vi "DHE_ParseAutoshutterCmd.vi"(8 "error in (no error)":errorcluster, 10 "argument":string, 11 "fd":i32) -> (0 "error out":errorcluster, 1 "ON?":bool, 2 "return value":i32, 3 "fd out":i32)   [LabVIEW 2016]
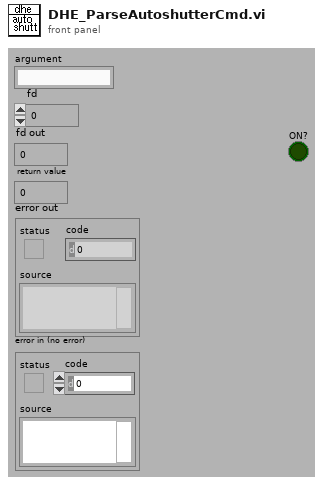
[diagram p1: front panel]
types:
  T1 = typedef "CMN_ContStatus.ctl" = cluster{"Response":string, "power":bool, "shutter":bool, "artifdata":bool, "idlemode":bool, "reset":bool, "gain":u8, "speed":u8, "resetPCI":bool, "autoshutter":bool, "TempSetPoint":i32, "multipleextensions":bool, "displayImage":bool, "coadding":bool, "images being coadded":i32, "Operation Mode":enum16{"normal", "coadd", "fawler"}, "frames to write":cluster{"subs":bool, "reset":bool, "exposed":bool}, "fawler samples":i32, "write auto":bool, "datatype":string, "frames to display":cluster{"subs":bool, "reset":bool, "exposed":bool}, "sur":i32, "autoclear":bool}
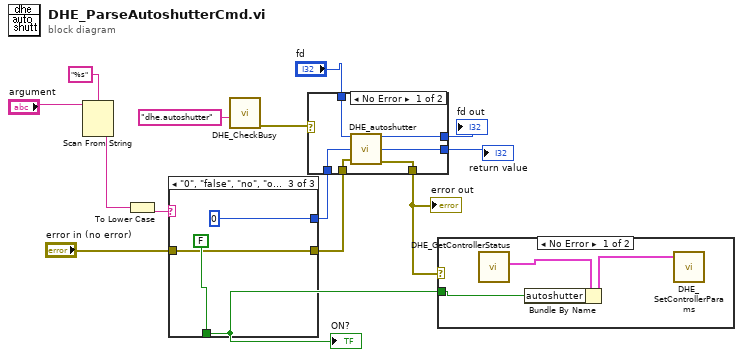
[diagram p0: block diagram]
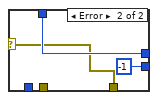
[diagram p2: hidden frame]
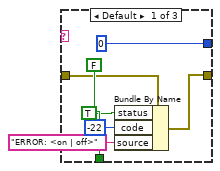
[diagram p4: hidden frame]
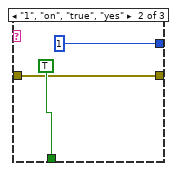
[diagram p5: hidden frame]
diagram:
  n1 = Scan From String(format string="%s" ("Format String"), input string="argument") -> (output 1=w13:string)  [unwired: 2 in, 4 out]
  n2 = To Lower Case(string=w13) -> (all lower case string=w11:string)
  n3 = case shown="\"0\", \"false\", \"no\", \"off\"" w11 {
    tunnel: [0 1 0] -> w12
    tunnel: [FALSE TRUE FALSE] -> w3
    tunnel: "error in (no error)" -> [w19 w22 w25]
    tunnel: [w15 w22 w25] -> w5
    frame Default {
      n4 = Bundle By Name(cluster=w19, "status"=TRUE, "code"=-22, "source"="ERROR: <on | off>") -> (w15:errorcluster)
    }
    frame "1", "on", "true", "yes" {
    }
    frame "0", "false", "no", "off" {
    }
  }
  "ON?" <- w3
  n5 = call "DHE_CheckBusy.vi"("command"="dhe.autoshutter") -> ("error out"=w2:errorcluster)  [unwired: 2 in, 8 out]
  n6 = case shown="No Error" w2 {
    selector: w2 -> [_ w34]
    tunnel: w12 -> [w33 _]
    tunnel: [w32 w36] -> w10
    tunnel: [w31 -1 ("return value")] -> w9
    tunnel: "fd" -> [w30 w36]
    tunnel: w5 -> [w29 _]
    tunnel: [w28 w34] -> w4
    frame No Error {
      n7 = call "DHE_autoshutter.vi"("fd"=w30, "flag"=w33, "error in (no error)"=w29) -> ("fd out"=w32:i32, "return value"=w31:i32, "error out"=w28:errorcluster)  [unwired: 10 out]
    }
    frame Error {
    }
  }
  "fd out" <- w10
  "return value" <- w9
  "error out" <- w4
  n8 = case shown="No Error" w4 {
    tunnel: w3 -> [w39 _]
    frame No Error {
      n9 = call "DHE_GetControllerStatus.vi"() -> ("ControllerStatus"=w38:T1)  [unwired: 11 out]
      n10 = Bundle By Name(cluster=w38, "autoshutter"=w39) -> (w37:T1)
      n11 = call "DHE_SetControllerParams.vi"("ControllerStatus"=w37) -> ()  [unwired: 1 in, 10 out]
    }
    frame Error {
    }
  }
